vi "video 00 simplest extraction.vi"() -> ()   [LabVIEW 2026]
panel:
  out "appended array":cluster{"output 7":dbl, "Instruction":string}[](array[cluster])
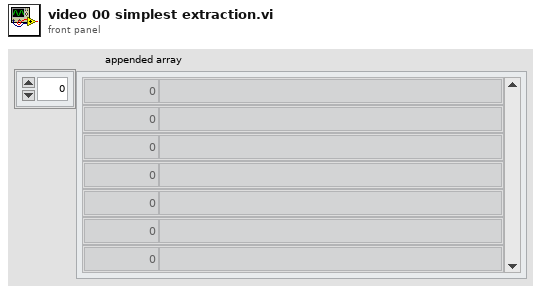
[diagram p1: front panel]
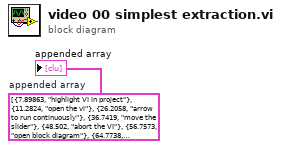
[diagram p0: block diagram]
diagram:
  w1 = cluster{"output 7":dbl, "Instruction":string}[] [{"output 7"=7.89863, "Instruction"="highlight VI in project"}, {"output 7"=11.2824, "Instruction"="open the vi"}, {"output 7"=26.2058, "Instruction"="arrow to run continuously"}, {"output 7"=36.7419, "Instruction"="move the slider"}, {"output 7"=48.502, "Instruction"="abort the VI"}, {"output 7"=56.7573, "Instruction"="open block diagram"}, {"output 7"=64.7738, "Instruction"="rearrange windows left right"}, {"output 7"=73.1166, "Instruction"="object highlight FP and BD elements"}, {"output 7"=91.6511, "Instruction"="object highlight wire"}, {"output 7"=142.766, "Instruction"="object highlight the dds"}, {"output 7"=145.111, "Instruction"="enable the diagram"}, {"output 7"=167.838, "Instruction"="run the vi"}, {"output 7"=176.318, "Instruction"="move the slider"}, {"output 7"=196.41, "Instruction"="objec higlight stop"}]  # appended array
  "appended array" <- w1
